vi "Signal Manipulation.vi"() -> ()   [LabVIEW 2023]
uses:
  <vilib>/Utility/error.llb/DialogType.ctl
panel:
  out "Difference":dbl
  out "Waveform Graph":dynamicdata(graph)
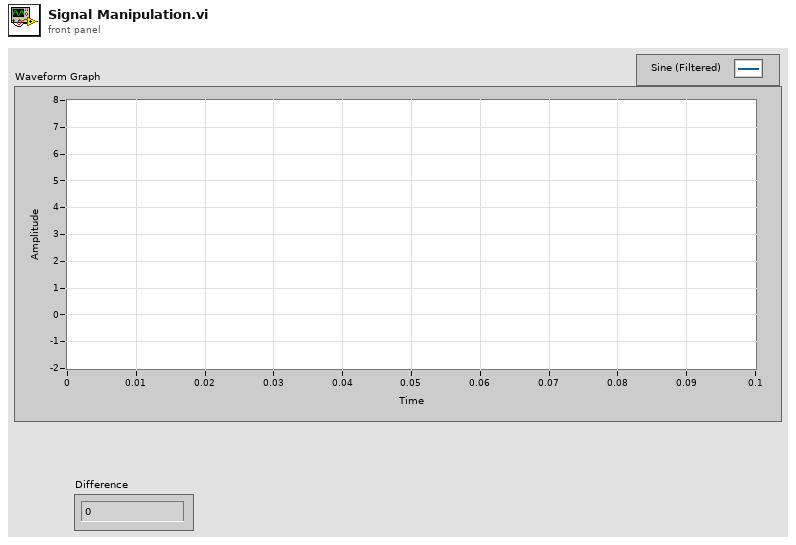
[diagram p1: front panel]
types:
  T1 = typedef "DialogType.ctl" = u16
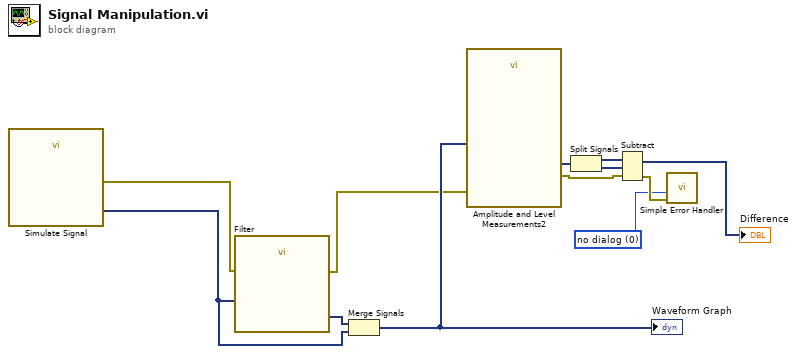
[diagram p0: block diagram]
diagram:
  w1 = T1 0 items=["no dialog", "OK message", "continue or stop message", "OK message + warnings", "continue/stop + warnings"] ("type of dialog (OK msg:1)")
  n1 = call "Simulate Signal"() -> ("Sine"=w11:dynamicdata, "error out"=w12:errorcluster)  [unwired: 14 in]
  n2 = call "Filter"("error in (no error)"=w12, "Signal"=w11) -> ("error out"=w4:errorcluster, "Filtered Signal"=w10:dynamicdata)  [unwired: 8 in]
  n3 = Merge Signals(w10, w11) -> (w9:dynamicdata)
  "Waveform Graph" <- w9
  n4 = call "Amplitude and Level Measurements2"("Signals"=w9, "error in (no error)"=w4) -> ("Peak to Peak"=w8:dynamicdata, "error out"=w3:errorcluster)  [unwired: 12 in]
  n5 = Split Signals(w8) -> (w7:dynamicdata, w6:dynamicdata)  [unwired: 2 in]
  n6 = Subtract(1:w6, 2:w7, 4:w3) -> (0:→"Difference":dynamicdata, 3:w2:errorcluster)
  n7 = call <vilib>:"Simple Error Handler.vi"("type of dialog (OK msg:1)"=w1, "error in (no error)"=w2) -> ()  [unwired: 3 in, 5 out]
